vi "Auto Match.vi"() -> ()   [LabVIEW 2018]
panel:
  out "반복 횟수":i32
  out "현재 값":u32 format="%#.0f"
  in  "일치하는 값":u32=50 max=1000 step=1
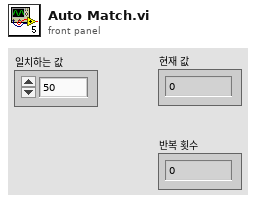
[diagram p1: front panel]
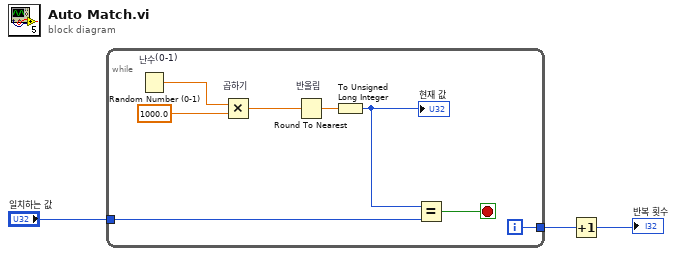
[diagram p0: block diagram]
diagram:
  n1 = while {
    tunnel: [w7] -> w3
    tunnel: "일치하는 값" -> [w6]
    i -> [w7]
    stop <- w8 stop-if-true
    n2 = Random Number (0-1) "난수(0-1)"() -> (number: 0 to 1=w11:dbl)
    n3 = Multiply "곱하기"(x=w11, y=1000.0) -> (x*y=w9:dbl)
    n4 = Round To Nearest "반올림"(number=w9) -> (nearest integer value=w5:dbl)
    n5 = To Unsigned Long Integer(number=w5) -> (unsigned 32bit integer=w4:u32)
    "현재 값" <- w4
    n6 = Equal?(x=w4, y=w6) -> (x = y?=w8:bool)
  }
  n7 = Increment(x=w3) -> (x+1=→"반복 횟수":i32)
